vi "calibrationSpectrometer_logEvent_MeasuredSpectrum.vi"(8 "error in (no error)":errorcluster, 11 "logevent_MeasuredSpectrum_Ctl":T1={"spectId"=0, "wavelength[2048]"=array[2048 elements], "intensity[2048]"=array[2048 elements], "imageName"="", "priority"=0}) -> (0 "error out":errorcluster, 2 "function return":i32, 3 "logevent_MeasuredSpectrum_Ctl out":T1)   [LabVIEW 2016, in "SALLV_calibrationSpectrometer.lvlib"]
doc: "int calibrationSpectrometer_shm_logEvent_MeasuredSpectrumLV(calibrationSpectrometer_logevent_MeasuredSpectrumLV *logevent_MeasuredSpectrum_Ctl );"
uses:
  SALLV_calibrationSpectrometer.lvlib
  DataTypes/logevent_MeasuredSpectrum.ctl
  SALLV_calibrationSpectrometer.so
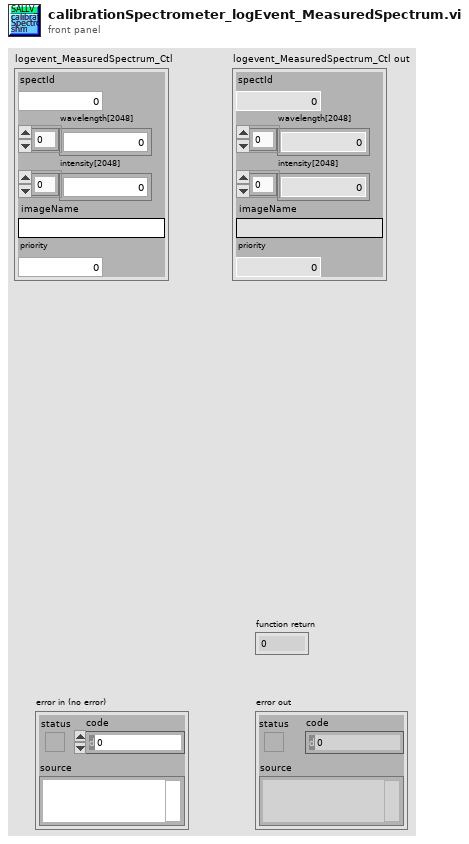
[diagram p1: front panel]
types:
  T1 = typedef "SALLV_calibrationSpectrometer.lvlib/logevent_MeasuredSpectrum.ctl" = cluster{"spectId":u16, "wavelength[2048]":dbl[], "intensity[2048]":dbl[], "imageName":string, "priority":i32}
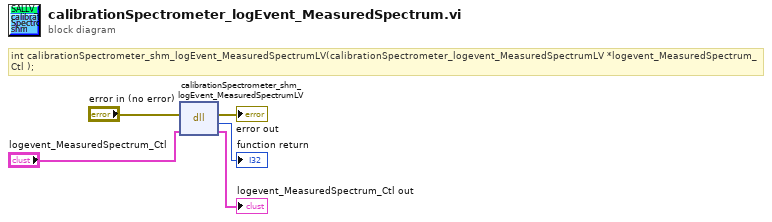
[diagram p0: block diagram]
diagram:
  # "int calibrationSpectrometer_shm_logEvent_MeasuredSpectrumLV(calibrationSpectrometer_logevent_MeasuredSpectrumLV *logevent_MeasuredSpectrum_Ctl );"
  n1 = dll-call lib="home/harini/TCS/sallv_sedspectrometer/SALLV_calibrationSpectrometer.*" fn="calibrationSpectrometer_shm_logEvent_MeasuredSpectrumLV"(error in="error in (no error)", "logevent_MeasuredSpectrum_Ctl"="logevent_MeasuredSpectrum_Ctl") -> (error out=→"error out":errorcluster, →"function return":i32, "logevent_MeasuredSpectrum_Ctl"=→"logevent_MeasuredSpectrum_Ctl out":T1)  [unwired: 2 in, 1 out]
